vi "Read Data File.vi"(0 "Filepath":path, 5 "Controller List":T2(array[cluster]), 7 "ValidFile?":bool, 11 "Error In":errorcluster) -> (1 "Gauge Number":string, 2 "Notes":string, 3 "TestCfgCluster":T3, 4 "Data":string[][](array[string]), 6 "Stats":string[][](array[string]), 8 "Profile":string[][](array[string]), 9 "TestStyle":string, 10 "Part#s":string[](array[string]), 12 "Cal Due Date":string, 14 "VoltLoc":string, 15 "Error Out":errorcluster)   [LabVIEW 2013]
uses:
  TypeDef/TestCfgCluster.ctl
  TypeDef/Controller Names.ctl
  <vilib>/Utility/file.llb/Write To Spreadsheet File (string).vi
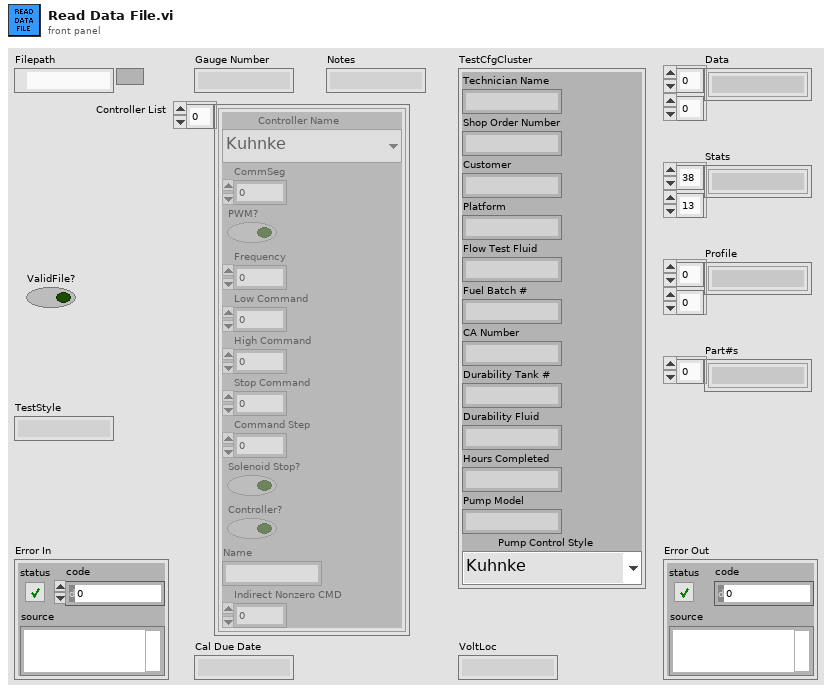
[diagram p1: front panel]
types:
  T1 = typedef "Controller Names.ctl" = enum16{"Kuhnke", "Helbako BLDC", "Conti", "Hella BLDC Screw", "Hella BLDC Turbine", "Helbako (old)", "TI PWM", "PSA", "Hella Gas", "Hella Diesel", "8 Comm", "10 Comm", "8 Comm Hella", "10 Comm Hella", "8 Comm Omron", "10 Comm Omron", "8 Comm Nissan", "10 Comm Nissan"}
  T2 = cluster{"Controller Name":T1, "CommSeg":i32, "PWM?":bool, "Frequency":i32, "Low Command":dbl, "High Command":dbl, "Stop Command":dbl, "Command Step":dbl, "Solenoid Stop?":bool, "Controller?":bool, "Name":string, "Indirect Nonzero CMD":dbl}[]
  T3 = typedef "TestCfgCluster.ctl" = cluster{"Technician Name":string, "Shop Order Number":string, "Customer":string, "Platform":string, "Flow Test Fluid":string, "Fuel Batch #":string, "CA Number":string, "Durability Tank #":string, "Durability Fluid":string, "Hours Completed":string, "Pump Model":string, "Pump Control Style":T1}
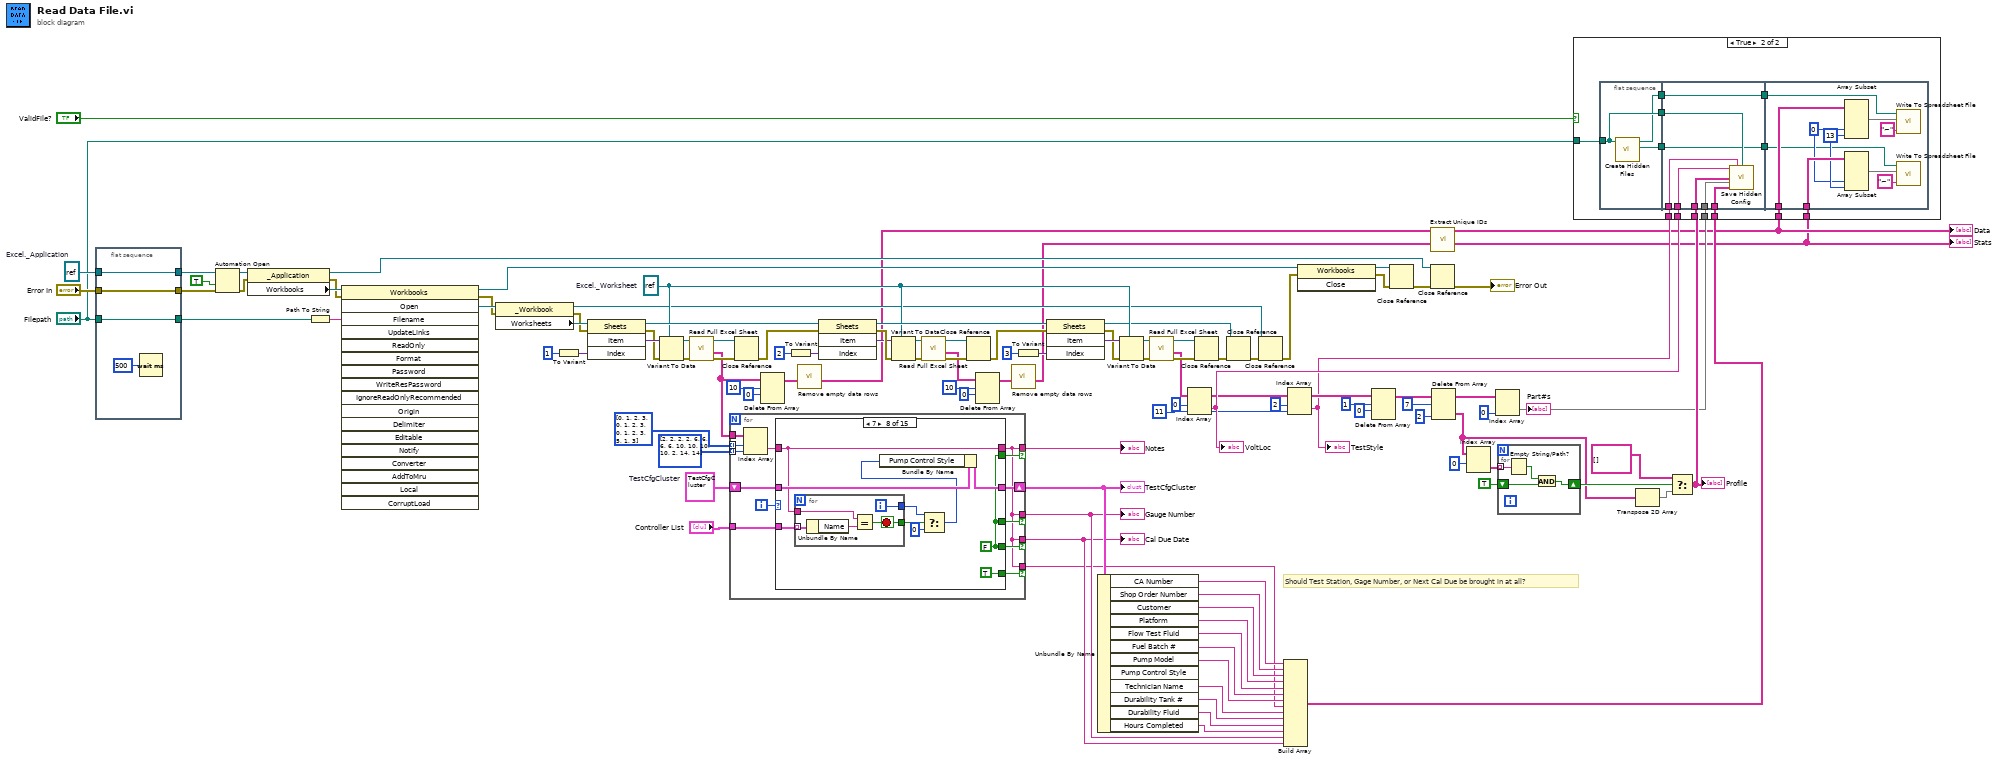
[diagram p0: block diagram]
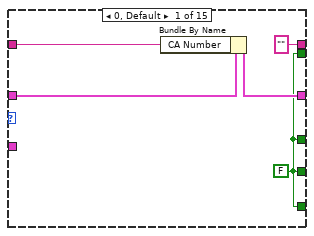
[diagram p3: hidden frame]
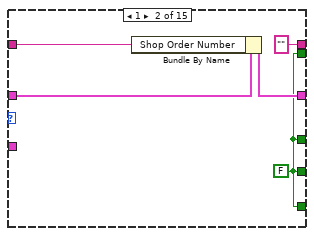
[diagram p4: hidden frame]
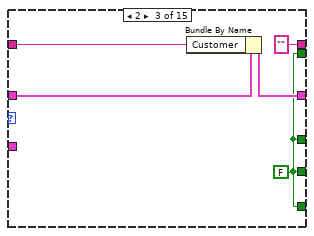
[diagram p5: hidden frame]
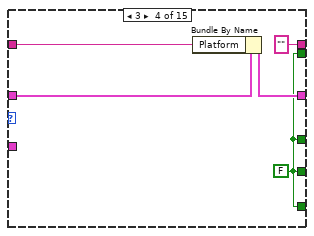
[diagram p6: hidden frame]
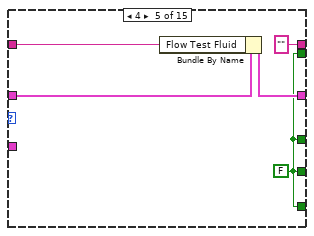
[diagram p7: hidden frame]
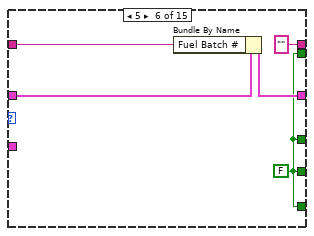
[diagram p8: hidden frame]
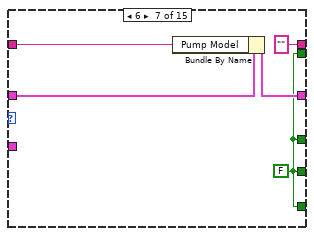
[diagram p9: hidden frame]
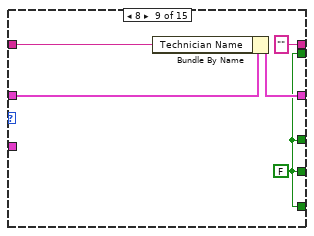
[diagram p10: hidden frame]
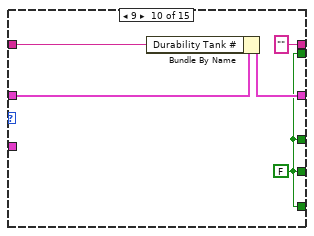
[diagram p11: hidden frame]
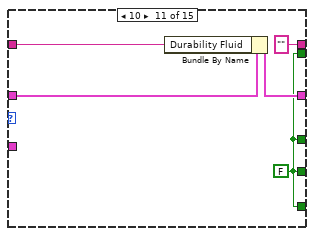
[diagram p12: hidden frame]
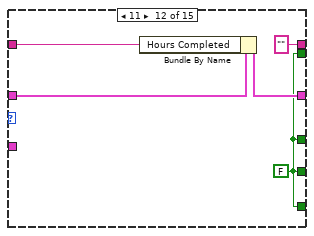
[diagram p13: hidden frame]
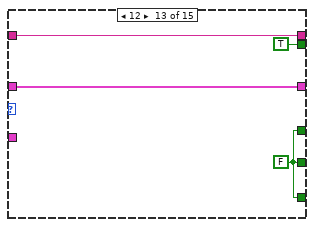
[diagram p14: hidden frame]
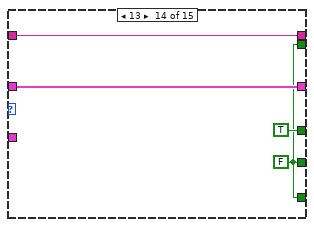
[diagram p15: hidden frame]
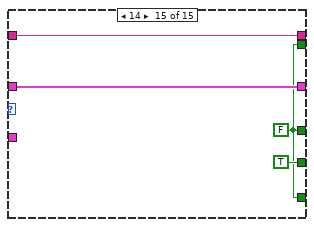
[diagram p16: hidden frame]
diagram:
  w9 = 11 ("disabled index (col)")
  w80 = T3 {"Technician Name"="", "Shop Order Number"="", "Customer"="", "Platform"="", "Flow Test Fluid"="", "Fuel Batch #"="", "CA Number"="", "Durability Tank #"="", "Durability Fluid"="", "Hours Completed"="", "Pump Model"="", "Pump Control Style"=enum."Kuhnke"}  # TestCfgCluster
  w85 = refnum<k7> refnum  # Excel._Worksheet
  w61 = refnum<k7> refnum  # Excel._Application
  # "Should Test Station, Gage Number, or Next Cal Due be brought in at all?"
  n1 = flat-sequence {
    tunnel: w61 -> [w114]
    tunnel: "Error In" -> [w115]
    tunnel: "Filepath" -> [w116]
    tunnel: [w116] -> w59
    tunnel: [w115] -> w58
    tunnel: [w114] -> w57
    frame #0 {
      n2 = Wait (ms)(milliseconds to wait=u32 500) -> ()  [unwired: 1 out]
    }
  }
  n3 = Automation Open(error in (no error)=w58, Automation Refnum=w57, 9:TRUE ("open new instance (false)")) -> (Automation Refnum=w110:refnum<k7>, error out=w111:errorcluster)  [unwired: 1 in]
  n4 = property class="_Application"(reference=w110, error in=w111) -> (reference out=w68:refnum<k7>, error out=w109:errorcluster, "Workbooks"=w112:refnum<k7>)
  n5 = Path To String(path=w59) -> (string=w108:string)
  n6 = invoke class="Workbooks" method="Open"(reference=w112, error in=w109, "Filename"=w108) -> (reference out=w66:refnum<k7>, error out=w69:errorcluster, "Open"=w70:refnum<k7>)  [unwired: 15 in, 15 out]
  n7 = property class="_Workbook"(reference=w70, error in=w69) -> (reference out=w81:refnum<k7>, error out=w105:errorcluster, "Worksheets"=w106:refnum<k7>)
  n8 = To Variant(anything=1) -> (Variant=w104:variant)
  n9 = invoke class="Sheets" method="Item"(reference=w106, error in=w105, "Index"=w104) -> (reference out=w89:refnum<k7>, error out=w102:errorcluster, "Item"=w103:variant)  [unwired: 1 in, 1 out]
  n10 = Variant To Data(error in=w102, type=w85, Variant=w103) -> (data=w100:refnum<k7>, error out=w101:errorcluster)
  n11 = call "Read Full Excel Sheet.vi"("Error In"=w101, "Excel._Worksheet"=w100) -> ("Error Out"=w99:errorcluster, "Data"=w76:string[][], "Reference Out"=w98:refnum<k7>)  [unwired: 7 in]
  n12 = for {
    tunnel: w76 -> [w129]
    shift-right: [w123] -> w27
    shift-left: w80 -> [w124]
    tunnel: i32[] [0, 1, 2, 3, 0, 1, 2, 3, 0, 1, 2, 3, 5, 1, 3] -> [w128] mode=indexing
    tunnel: i32[] [2, 2, 2, 2, 6, 6, 6, 6, 10, 10, 10, 10, 2, 14, 14] -> [w127] mode=indexing
    tunnel: [w117] -> w77 if=w122
    tunnel: [w117] -> w15 if=w121
    tunnel: [w117] -> w14 if=w120
    tunnel: "Controller List" -> [w119]
    tunnel: [w117] -> w1 if=w118
    i -> [w126]
    n13 = Index Array(array=w129, index (row)=w128, index (col)=w127) -> (element=w125:string)
    n14 = case shown="7" w126 {
      tunnel: w125 -> [w134 w139 w144 w149 w154 w159 w164 w165 w184 w189 w194 w196 w202 w206 w210]
      tunnel: w124 -> [w133 w138 w143 w148 w153 w158 w163 w174 w183 w188 w193 w199 w203 w207 w211]
      tunnel: [w132 w137 w142 w147 w152 w157 w162 w173 w182 w187 w192 w198 w203 w207 w211] -> w123
      tunnel: ["" ("String") "" ("String") "" ("String") "" ("String") "" ("String") "" ("String") "" ("String") w165 "" ("String") "" ("String") "" ("String") "" ("String") w202 w206 w210] -> w117
      tunnel: [w130 w135 w140 w145 w150 w155 w160 w172 w180 w185 w190 w195 TRUE w204 w208] -> w122
      tunnel: [w130 w135 w140 w145 w150 w155 w160 w172 w180 w185 w190 w195 w200 TRUE w208] -> w121
      tunnel: [w130 w135 w140 w145 w150 w155 w160 w172 w180 w185 w190 w195 w200 w204 TRUE] -> w120
      tunnel: w119 -> [_ _ _ _ _ _ _ w171 _ _ _ _ _ _ _]
      tunnel: [w130 w135 w140 w145 w150 w155 w160 TRUE w180 w185 w190 w195 w200 w204 w208] -> w118
      frame 0, Default {
        w130 = FALSE
        n15 = Bundle By Name(cluster=w133, "CA Number"=w134) -> (w132:T3)
      }
      frame 1 {
        w135 = FALSE
        n16 = Bundle By Name(cluster=w138, "Shop Order Number"=w139) -> (w137:T3)
      }
      frame 2 {
        w140 = FALSE
        n17 = Bundle By Name(cluster=w143, "Customer"=w144) -> (w142:T3)
      }
      frame 3 {
        w145 = FALSE
        n18 = Bundle By Name(cluster=w148, "Platform"=w149) -> (w147:T3)
      }
      frame 4 {
        w150 = FALSE
        n19 = Bundle By Name(cluster=w153, "Flow Test Fluid"=w154) -> (w152:T3)
      }
      frame 5 {
        w155 = FALSE
        n20 = Bundle By Name(cluster=w158, "Fuel Batch #"=w159) -> (w157:T3)
      }
      frame 6 {
        w160 = FALSE
        n21 = Bundle By Name(cluster=w163, "Pump Model"=w164) -> (w162:T3)
      }
      frame 7 {
        w172 = FALSE
        n22 = for {
          tunnel: w165 -> [w178]
          tunnel: w171 -> [w179] mode=indexing
          tunnel: [w176] -> w169
          tunnel: [w175] -> w170
          i -> [w176]
          stop <- w175 stop-if-true
          n23 = Unbundle By Name(w179) -> ("Name"=w177:string)
          n24 = Equal?(x=w178, y=w177) -> (x = y?=w175:bool)
        }
        n25 = Select(t=w169, s=w170, f=0) -> (s? t:f=w166:i32)
        n26 = Bundle By Name(cluster=w174, "Pump Control Style"=w166) -> (w173:T3)
      }
      frame 8 {
        w180 = FALSE
        n27 = Bundle By Name(cluster=w183, "Technician Name"=w184) -> (w182:T3)
      }
      frame 9 {
        w185 = FALSE
        n28 = Bundle By Name(cluster=w188, "Durability Tank #"=w189) -> (w187:T3)
      }
      frame 10 {
        w190 = FALSE
        n29 = Bundle By Name(cluster=w193, "Durability Fluid"=w194) -> (w192:T3)
      }
      frame 11 {
        w195 = FALSE
        n30 = Bundle By Name(cluster=w199, "Hours Completed"=w196) -> (w198:T3)
      }
      frame 12 {
        w200 = FALSE
      }
      frame 13 {
        w204 = FALSE
      }
      frame 14 {
        w208 = FALSE
      }
    }
  }
  "Notes" <- w77
  "TestCfgCluster" <- w27
  "Gauge Number" <- w15
  "Cal Due Date" <- w14
  n31 = Close Reference(reference=w98, error in (no error)=w99) -> (error out=w86:errorcluster)
  n32 = Delete From Array(array=w76, length=10, index (row)=0) -> (array with subset deleted=w34:string[][])  [unwired: 1 in, 1 out]
  n33 = To Variant(anything=2) -> (Variant=w91:variant)
  n34 = call "Remove empty data rows.vi"("Array In"=w34) -> ("Array Out"=w6:string[][])  [unwired: 10 in]
  n35 = invoke class="Sheets" method="Item"(reference=w89, error in=w86, "Index"=w91) -> (reference out=w88:refnum<k7>, error out=w93:errorcluster, "Item"=w92:variant)  [unwired: 1 in, 1 out]
  n36 = Variant To Data(error in=w93, type=w85, Variant=w92) -> (data=w95:refnum<k7>, error out=w94:errorcluster)
  n37 = call "Read Full Excel Sheet.vi"("Error In"=w94, "Excel._Worksheet"=w95) -> ("Error Out"=w96:errorcluster, "Data"=w71:string[][], "Reference Out"=w97:refnum<k7>)  [unwired: 7 in]
  n38 = Close Reference(reference=w97, error in (no error)=w96) -> (error out=w87:errorcluster)
  n39 = Delete From Array(array=w71, length=10, index (row)=0) -> (array with subset deleted=w33:string[][])  [unwired: 1 in, 1 out]
  n40 = call "Remove empty data rows.vi"("Array In"=w33) -> ("Array Out"=w5:string[][])  [unwired: 10 in]
  n41 = To Variant(anything=3) -> (Variant=w55:variant)
  n42 = invoke class="Sheets" method="Item"(reference=w88, error in=w87, "Index"=w55) -> (reference out=w82:refnum<k7>, error out=w53:errorcluster, "Item"=w54:variant)  [unwired: 1 in, 1 out]
  n43 = Unbundle By Name(w27) -> ("CA Number"=w26:string, "Shop Order Number"=w25:string, "Customer"=w24:string, "Platform"=w23:string, "Flow Test Fluid"=w22:string, "Fuel Batch #"=w21:string, "Pump Model"=w20:string, "Technician Name"=w19:string, "Durability Tank #"=w18:string, "Durability Fluid"=w17:string, "Hours Completed"=w16:string)  [unwired: 1 out]
  n44 = Variant To Data(error in=w53, type=w85, Variant=w54) -> (data=w51:refnum<k7>, error out=w52:errorcluster)
  n45 = call "Read Full Excel Sheet.vi"("Error In"=w52, "Excel._Worksheet"=w51) -> ("Error Out"=w50:errorcluster, "Data"=w10:string[][], "Reference Out"=w49:refnum<k7>)  [unwired: 7 in]
  n46 = Index Array(array=w10, index (row)=0, index (col)=w9) -> (element=w30:string)
  "VoltLoc" <- w30
  n47 = Close Reference(reference=w49, error in (no error)=w50) -> (error out=w84:errorcluster)
  n48 = Close Reference(reference=w82, error in (no error)=w84) -> (error out=w83:errorcluster)
  n49 = Close Reference(reference=w81, error in (no error)=w83) -> (error out=w64:errorcluster)
  n50 = Build Array(w26, w25, w24, w23, w22, w21, w20, w1, w19, w18, w17, w16, w15, w14) -> (w13:string[])
  n51 = Index Array(array=w10, index (row)=2, index (col)=w9) -> (element=w7:string)
  "TestStyle" <- w7
  n52 = invoke class="Workbooks" method="Close"(reference=w66, error in=w64) -> (reference out=w62:refnum<k7>, error out=w63:errorcluster)  [unwired: 1 in, 1 out]
  n53 = Delete From Array(array=w10, length=1, index (row)=0) -> (array with subset deleted=w45:string[][])  [unwired: 1 in, 1 out]
  n54 = Close Reference(reference=w62, error in (no error)=w63) -> (error out=w65:errorcluster)
  n55 = call "Extract Unique IDs.vi"("Stats"=w5, "Data"=w6) -> ("Stats with IDs"=w3:string[][], "Data with IDs"=w4:string[][])  [unwired: 8 in]
  "Data" <- w4
  "Stats" <- w3
  n56 = Close Reference(reference=w68, error in (no error)=w65) -> (error out=→"Error Out":errorcluster)
  n57 = Delete From Array(array=w45, length=7, index (col)=2 ("disabled index (col)")) -> (deleted portion=w11:string[][], array with subset deleted=w42:string[][])  [unwired: 1 in]
  n58 = Index Array(array=w11, index (row)=0) -> (element=w40:string[])  [unwired: 1 in]
  n59 = Index Array(array=w42, index (col)=0 ("disabled index (col)")) -> (element=w28:string[])  [unwired: 1 in]
  "Part#s" <- w28
  n60 = for {
    tunnel: w40 -> [w215] mode=indexing
    shift-right: [w213] -> w37
    shift-left: TRUE -> [w212]
    n61 = Empty String/Path?(string/path=w215) -> (empty?=w214:bool)
    n62 = And(x=w214, y=w212) -> (x .and. y?=w213:bool)
  }
  n63 = Transpose 2D Array(2D array=w11) -> (transposed array=w35:string[][])
  n64 = Select(t=string[][] [], s=w37, f=w35) -> (s? t:f=w29:string[][])
  "Profile" <- w29
  n65 = case shown="True" "ValidFile?" {
    tunnel: "Filepath" -> [_ w228]
    tunnel: w30 -> [_ w226]
    tunnel: w29 -> [_ w225]
    tunnel: w28 -> [_ w224]
    tunnel: w13 -> [_ w223]
    tunnel: w3 -> [_ w222]
    tunnel: w4 -> [_ w221]
    tunnel: w7 -> [_ w216]
    frame False {
    }
    frame True {
      n66 = flat-sequence {
        tunnel: w228 -> [w231]
        tunnel: [w231] -> w227
        tunnel: [w230] -> w219
        tunnel: [w229] -> w217
        tunnel: w227 -> [w239]
        tunnel: w226 -> [w238]
        tunnel: w225 -> [w237]
        tunnel: w224 -> [w236]
        tunnel: w223 -> [w235]
        tunnel: [w234] -> w220
        tunnel: w219 -> [w234]
        tunnel: [w233] -> w218
        tunnel: w217 -> [w233]
        tunnel: w216 -> [w232]
        tunnel: w222 -> [w245]
        tunnel: w221 -> [w244]
        tunnel: w220 -> [w241]
        tunnel: w218 -> [w240]
        frame #0 {
          n67 = call "Create Hidden Files.vi"("DataFilePath"=w231) -> ("Stats path"=w229:path, "Data Path"=w230:path)  [unwired: 8 in, 1 out]
        }
        frame #1 {
          n68 = call "Save Hidden Config.vi"("EnumV"=w238, "EnumRadio"=w232, "DataFilePath"=w239, "Profile"=w237, "Serial Numbers"=w236, "Header Info"=w235) -> ()  [unwired: 10 in]
        }
        frame #2 {
          w243 = 13 ("length")
          w242 = 0 ("index")
          n69 = Array Subset(array=w244, index (col)=w242, length (col)=w243) -> (w249:string[][])  [unwired: 2 in]
          n70 = Array Subset(array=w245, index (col)=w242, length (col)=w243) -> (w247:string[][])  [unwired: 2 in]
          n71 = call-poly <vilib>:"Write To Spreadsheet File.vi"("delimiter (\\t)"="~" ("delimiter (\\t)"), "2D data"=w249, "file path (dialog if empty)"=w241) -> ()  [unwired: 5 in, 1 out]
          n72 = call-poly <vilib>:"Write To Spreadsheet File.vi"("delimiter (\\t)"="~" ("delimiter (\\t)"), "2D data"=w247, "file path (dialog if empty)"=w240) -> ()  [unwired: 5 in, 1 out]
        }
      }
    }
  }
